vi "Close-session.vi"(8 "error in (no error)":errorcluster, 11 "Camera in":refnum<class "Camera.lvclass">) -> (0 "error out":errorcluster, 2 "IMAQ Session":refnum<k11>, 3 "Camera out":refnum<class "Camera.lvclass">, 5 "Success?":bool=TRUE)   [LabVIEW 2013, in "CameraVision.lvlib" / "Camera.lvclass"]
uses:
  Camera.lvclass
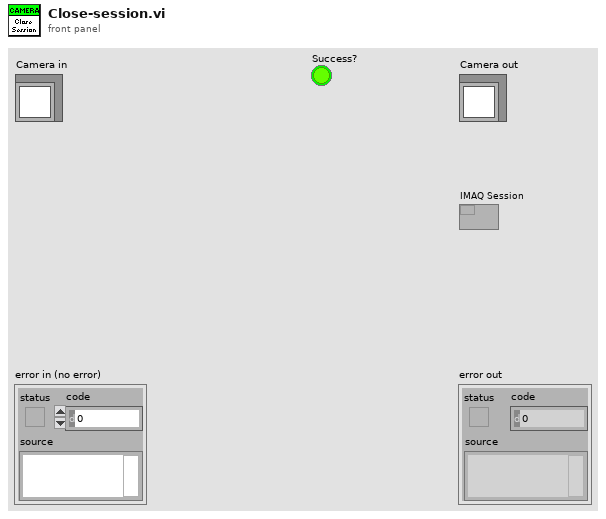
[diagram p1: front panel]
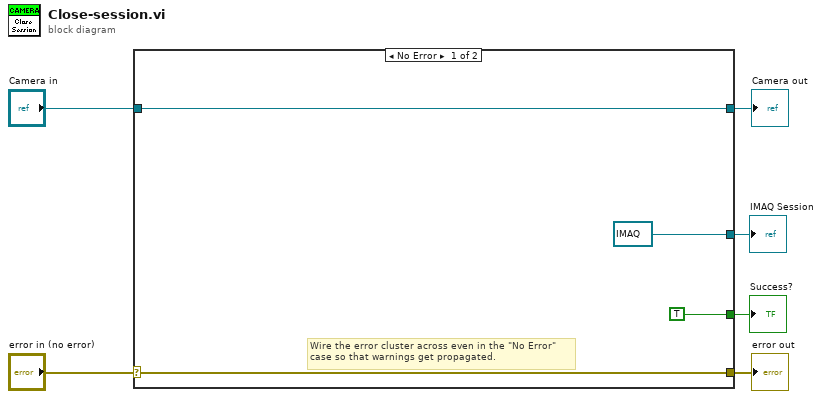
[diagram p0: block diagram]
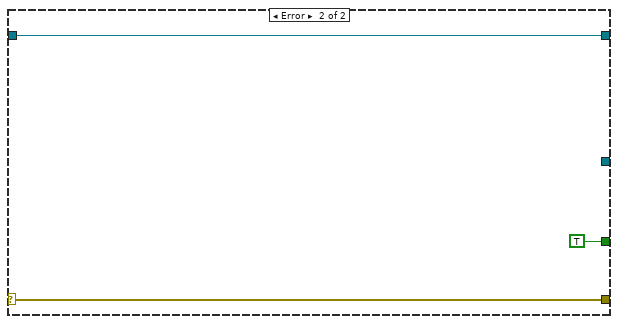
[diagram p2: hidden frame]
diagram:
  n1 = case shown="No Error" "error in (no error)" {
    selector: "error in (no error)" -> [w9 w13]
    tunnel: [w9 w13] -> w5
    tunnel: [w10 w12] -> w3
    tunnel: "Camera in" -> [w10 w12]
    tunnel: [refnum<k11> refnum ("IMAQ Session Out") _] -> w2
    tunnel: [TRUE TRUE] -> w1
    frame No Error {
      # "Wire the error cluster across even in the \"No Error\"\ncase so that warnings get propagated."
    }
    frame Error {
    }
  }
  "error out" <- w5
  "Camera out" <- w3
  "IMAQ Session" <- w2
  "Success?" <- w1
